vi "saveImages.vi"(8 "error in (no error)":errorcluster, 10 "Array":path[](array[path]), 11 "Camera in":refnum<class "Camera.lvclass">) -> (0 "error out":errorcluster, 3 "Camera out":refnum<class "Camera.lvclass">)   [LabVIEW 2009, in "Hardware.lvlib" / "Channels.lvlib" / "Camera.lvclass"]
uses:
  Camera.lvclass
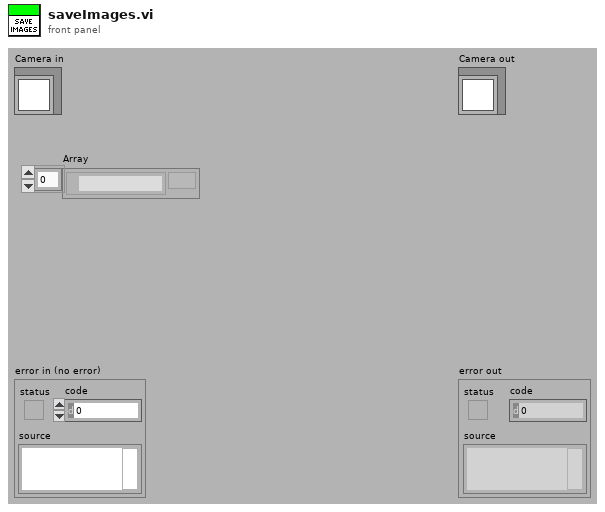
[diagram p1: front panel]
types:
  T1 = typedef "IMAQ Image.ctl" = refnum<image>
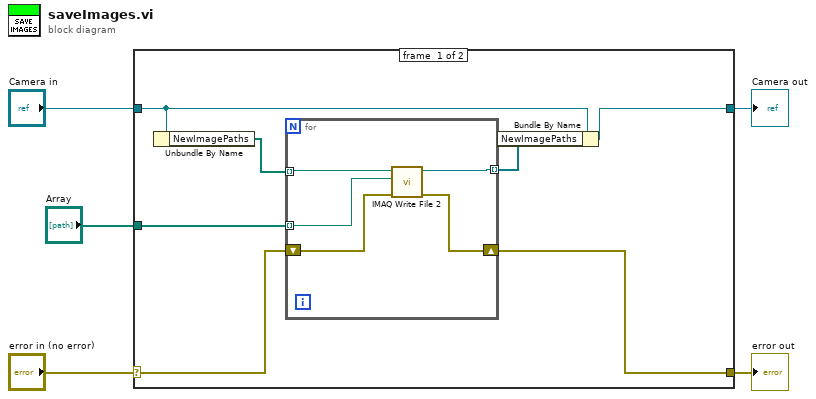
[diagram p0: block diagram]
diagram:
  n1 = case shown="No Error" "error in (no error)" {
    selector: "error in (no error)" -> [w10 w19]
    tunnel: [w9 w19] -> w4
    tunnel: [w6 w18] -> w2
    tunnel: "Camera in" -> [w7 w18]
    tunnel: "Array" -> [w11 _]
    frame #0 {
      n2 = Unbundle By Name(w7) -> ("NewImagePaths"=w12:path[])
      n3 = for {
        tunnel: w12 -> [w17] mode=indexing
        tunnel: w11 -> [w16] mode=indexing
        shift-right: [w14] -> w9
        shift-left: w10 -> [w15]
        tunnel: [w13] -> w8 mode=indexing
        n4 = call-poly "IMAQ Write File 2"("error in (no error)"=w15, "File Path"=w16, "Image"=w17) -> ("error out"=w14:errorcluster, "Image Out (duplicate)"=w13:T1)  [unwired: 7 in]
      }
      n5 = Bundle By Name(cluster=w7, "NewImagePaths"=w8) -> (w6:refnum<class "Camera.lvclass">)
    }
    frame #1 {
    }
  }
  "error out" <- w4
  "Camera out" <- w2
